vi "init_commands.vi"(8 "error in (no error)":errorcluster caption="错误输入（无错误）", 11 "OneMotion 输入":refnum<class "OneMotion.lvclass">) -> (0 "error out":errorcluster caption="错误输出", 3 "OneMotion 输出":refnum<class "OneMotion.lvclass">)   [LabVIEW 2016, in "MotionControl.lvlib" / "OneMotion.lvclass"]
uses:
  <userlib>/MotionControl/OneMotion/OneMotion.lvclass
  <userlib>/MotionControl/OneMotion/cmd_motion.ctl
  <userlib>/MotionControl/OneMotion/OneMotion.lvclass/OneMotion.ctl
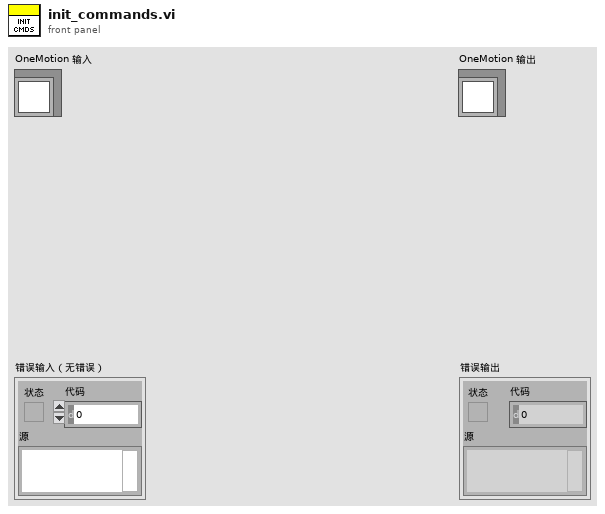
[diagram p1: front panel]
types:
  T1 = typedef "MotionControl.lvlib/OneMotion.lvclass/cmd_motion.ctl" = enum16{"NONE", "MOVE_MOTION", "EXIT", "STP_MOTION", "SPEED_MOTION", "WAIT_FOR_S3", "WAIT_A_TIME", "SKIP"}
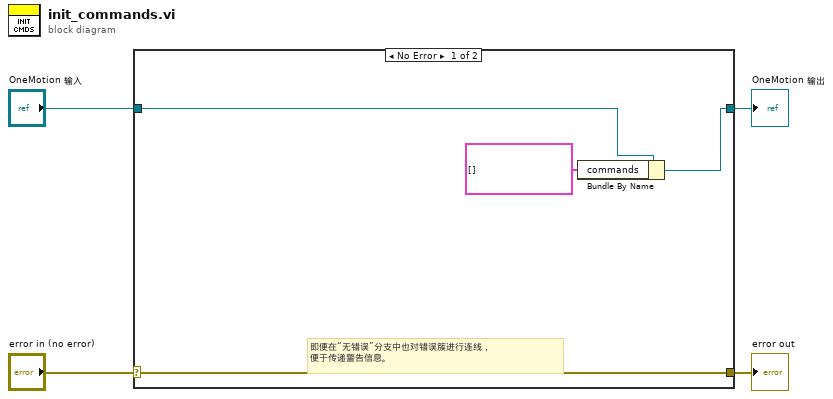
[diagram p0: block diagram]
diagram:
  n1 = case shown="No Error" "error in (no error)" {
    selector: "error in (no error)" -> [w8 w10]
    tunnel: [w8 w10] -> w3
    tunnel: [w6 w9] -> w1
    tunnel: "OneMotion 输入" -> [w7 w9]
    frame No Error {
      # "即便在“无错误”分支中也对错误簇进行连线，\n便于传递警告信息。"
      n2 = Bundle By Name(cluster=w7, "commands"=cluster{"cmd":T1, "cmd data":variant}[] []) -> (w6:refnum<class "OneMotion.lvclass">)
    }
    frame Error {
    }
  }
  "error out" <- w3
  "OneMotion 输出" <- w1
